vi "camera start acquire - subvi.vi"(1 "error in":errorcluster) -> (0 "error out":errorcluster)   [LabVIEW 2014]
doc: "Starts an iXon acquisition (if not already running)"
uses:
  Library Files - Andor and MadCity/Andorlib/atmcd32d.lvlib
panel:
  out "function return":u32
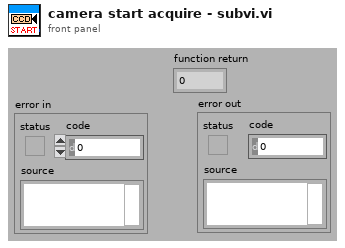
[diagram p1: front panel]
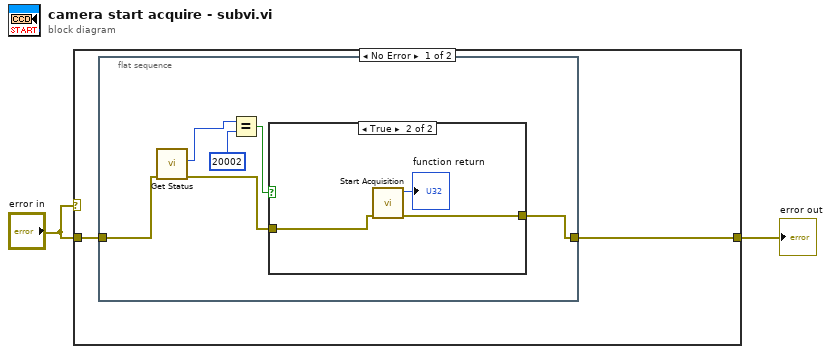
[diagram p0: block diagram]
diagram:
  n1 = case shown="No Error" "error in" {
    tunnel: "error in" -> [w3 w15]
    tunnel: [w4 w15] -> w2
    frame No Error {
      n2 = flat-sequence {
        tunnel: [w9] -> w4
        tunnel: w3 -> [w8]
        frame #0 {
          n3 = call "Get Status.vi"("error in (no error)"=w8) -> ("error out"=w10:errorcluster, "function return"=w5:u32)  [unwired: 8 in, 1 out]
          n4 = Equal?(x=w5, y=20002) -> (x = y?=w6:bool)
          n5 = case shown="True" w6 {
            tunnel: w10 -> [w11 w14]
            tunnel: [w11 w13] -> w9
            frame False {
            }
            frame True {
              n6 = call "Start Acquisition.vi"("error in (no error)"=w14) -> ("error out"=w13:errorcluster, "function return"=→"function return":u32)  [unwired: 9 in]
            }
          }
        }
      }
    }
    frame Error {
    }
  }
  "error out" <- w2
